vi "pulsed_counts-2017.07.10.vi"(0 "Commands":T1(array[cluster]) {"Time" format="%.3p"; "Op Code" items=["Continue", "Stop", "Loop", "End Loop", "JSR", "RTS", "Branch", "Long Delay", "Wait"]}, 5 "T1_parameters":T2={"pulse_period_us"=100.0, "pulse_width_us"=50.0, "read_delay_us"=0.0, "read_width_us"=1.0, "repetitions"=0} {"read_width_us" min=0.0 max=1000.0 format="%#_6f"; "pulse_period_us" format="%#_6p"}) -> (4 "mean_qPhotons":dbl, 6 "timetags":u32[](graph))   [LabVIEW 2014]
uses:
  <vilib>/DAQmx/read.llb/DAQmx Read (Counter 1D U32 1Chan NSamp).vi
panel:
  out "q_reads":i32
  out "Waveform Chart 4":u32[][](graph)
  # "1"
  # "2"
  # "3"
  # "4"
  # "5"
  # "6"
  # "7"
  # "8"
  # "9"
  # "10"
  # "11"
  # "12"
  # "13"
  # "14"
  # "15"
  # "16"
  # "17"
  # "18"
  # "19"
  # "20"
  # "21"
  # "22"
  # "23"
  # "24"
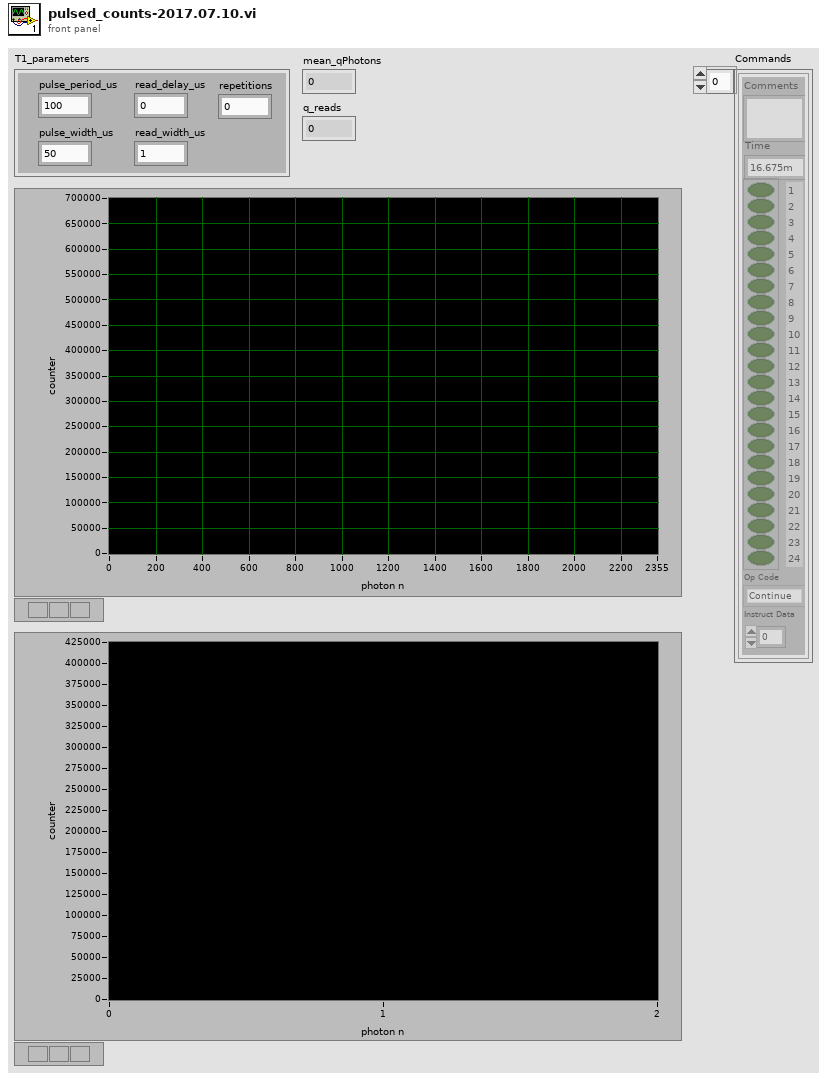
[diagram p1: front panel]
types:
  T1 = cluster{"Instruct Data":i32, "Op Code":i32, "Flags":bool[], "Comments":string, "Time":dbl}[]
  T2 = cluster{"pulse_period_us":dbl, "pulse_width_us":dbl, "read_delay_us":dbl, "read_width_us":dbl, "repetitions":i32}
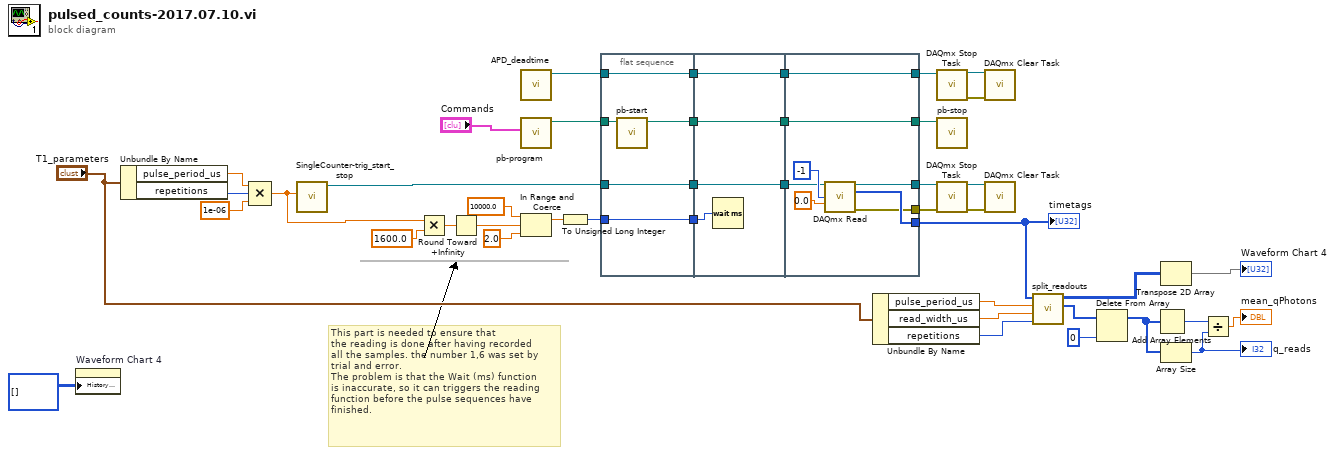
[diagram p0: block diagram]
diagram:
  # "This part is needed to ensure that\nthe reading is done after having recorded\nall the samples. the number 1,6 was set by\ntrial and error. \nThe problem is that the Wait (ms) function \nis inaccurate, so it can triggers the reading\nfunction before the pulse sequences have\nfinished."
  n1 = property on="Waveform Chart 4" class="WFChart (strict)"("History Data"=u32[][] []) -> ()  [unwired: 2 in, 2 out]
  n2 = Unbundle By Name("T1_parameters") -> ("pulse_period_us"=w39:dbl, "repetitions"=w38:i32)
  n3 = Compound Arithmetic op=MULTIPLY(w39, w38, 1e-06 ("y")) -> (w36:dbl)
  n4 = call "SingleCounter-trig_start_stop.vi"("Duration_s"=w36) -> ("task out"=w40:refnum<k21>)  [unwired: 8 in, 2 out]
  n5 = Multiply(x=w36, y=1600.0) -> (x*y=w8:dbl)
  n6 = Round Toward +Infinity(x=w8) -> (ceil(x): smallest int >= x=w7:dbl)
  n7 = call "APD_deadtime.vi"() -> ("filtered APD"=w24:refnum<k21>)  [unwired: 6 in, 1 out]
  n8 = call "pb-program.vi"("Commands"="Commands") -> ("path out"=w18:path)  [unwired: 10 in]
  n9 = In Range and Coerce(upper limit=10000.0, x=w7, lower limit=2.0) -> (coerced(x)=w33:dbl)  [unwired: 1 out]
  n10 = To Unsigned Long Integer(number=w33) -> (unsigned 32bit integer=w32:u32)
  n11 = flat-sequence {
    tunnel: w24 -> [w47]
    tunnel: w32 -> [w48]
    tunnel: w40 -> [w49]
    tunnel: [w49] -> w21
    tunnel: [w48] -> w20
    tunnel: [w47] -> w19
    tunnel: w18 -> [w46]
    tunnel: [w45] -> w15
    tunnel: [w53] -> w34
    tunnel: [w51] -> w25
    tunnel: w21 -> [w53]
    tunnel: w20 -> [w52]
    tunnel: w19 -> [w51]
    tunnel: [w50] -> w16
    tunnel: w15 -> [w50]
    tunnel: [w60] -> w28
    tunnel: w34 -> [w59]
    tunnel: [w57] -> w23
    tunnel: w25 -> [w57]
    tunnel: [w56] -> w17
    tunnel: w16 -> [w56]
    tunnel: [w55] -> w14
    tunnel: [w54] -> w9
    frame #0 {
      n12 = call "pb-start.vi"("path in"=w46) -> ("path out"=w45:path)  [unwired: 10 in]
    }
    frame #1 {
      n13 = Wait (ms)(milliseconds to wait=w52) -> ()  [unwired: 1 out]
    }
    frame #2 {
      n14 = call-poly <vilib>:"DAQmx Read.vi"("task/channels in"=w59, "number of samples per channel"=-1, "timeout"=0.0) -> ("task out"=w55:refnum<k21>, "data"=w60:u32[], "error out"=w54:errorcluster)  [unwired: 10 in]
    }
  }
  n15 = Unbundle By Name("T1_parameters") -> ("pulse_period_us"=w27:dbl, "read_width_us"=w13:dbl, "repetitions"=w26:i32)
  n16 = call <vilib>:"DAQmx Stop Task.vi"("task/channels in"=w23) -> ("task out"=w42:refnum<k21>, "error out"=w41:errorcluster)  [unwired: 13 in]
  n17 = call "pb-stop.vi"("path in"=w17) -> ()  [unwired: 9 in, 2 out]
  n18 = call <vilib>:"DAQmx Stop Task.vi"("task/channels in"=w14, "error in"=w9) -> ("task out"=w44:refnum<k21>, "error out"=w43:errorcluster)  [unwired: 12 in]
  n19 = call <vilib>:"DAQmx Clear Task.vi"("task in"=w42, "error in"=w41) -> ()  [unwired: 13 in, 1 out]
  n20 = call <vilib>:"DAQmx Clear Task.vi"("task in"=w44, "error in"=w43) -> ()  [unwired: 13 in, 1 out]
  n21 = call "split_readouts.vi"("repetitions"=w26, "read_width_us"=w13, "pulse_period_us"=w27, "timetags"=w28) -> ("q_photons"=w3:i32[], "readouts"=w22:u32[][])  [unwired: 6 in]
  n22 = Delete From Array(array=w3, index=0) -> (array with subset deleted=w5:i32[])  [unwired: 1 in, 1 out]
  n23 = Add Array Elements(numeric array=w5) -> (sum=w12:i32)
  n24 = Transpose 2D Array(2D array=w22) -> (transposed array=→"Waveform Chart 4":u32[][])
  n25 = Array Size(array=w5) -> (size(s)=w11:i32)
  "q_reads" <- w11
  n26 = Divide(x=w12, y=w11) -> (x/y=→"mean_qPhotons":dbl)
  "timetags" <- w28
